vi "Divide Speed.vi"(0 "Reset":bool, 3 "Speed":bool, 4 "Y":dbl, 5 "X":dbl) -> (1 "Yout":dbl, 2 "Xout":dbl)   [LabVIEW 2016]
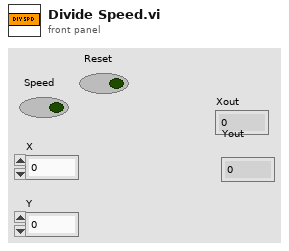
[diagram p1: front panel]
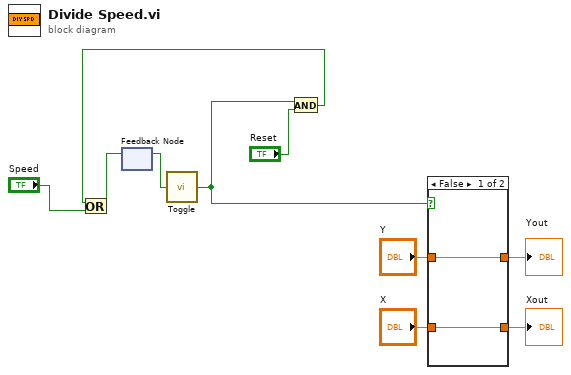
[diagram p0: block diagram]
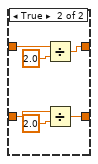
[diagram p2: hidden frame]
diagram:
  n1 = feedback #1() -> (w3:bool)  [unwired: 1 in]
  n2 = call "Toggle.vi"("Input"=w3) -> ("Output"=w6:bool)  [unwired: 4 in]
  n3 = And(x=w6, y="Reset") -> (x .and. y?=w2:bool)
  n4 = Or(x=w2, y="Speed") -> (x .or. y?=w4:bool)
  n5 = feedback-in #1(w4) -> ()
  n6 = case shown="False" w6 {
    tunnel: "Y" -> [w12 w18]
    tunnel: "X" -> [w11 w15]
    tunnel: [w11 w14] -> w8
    tunnel: [w12 w13] -> w7
    frame False {
    }
    frame True {
      n7 = Divide(x=w18, y=2.0) -> (x/y=w13:dbl)
      n8 = Divide(x=w15, y=2.0) -> (x/y=w14:dbl)
    }
  }
  "Xout" <- w8
  "Yout" <- w7
